vi "Start Async.vi"(8 "error in":errorcluster, 11 "gRPC Server in":refnum<class "ServiceBase.lvclass">) -> (0 "error out":errorcluster, 3 "gRPC Server out":refnum<class "ServiceBase.lvclass">)   [LabVIEW 2020, in "gRPC-servicer-release.lvlib" / "ServiceBase.lvclass"]
uses:
  gRPC Data Server Engine Windows.llb/ServiceBase.lvclass
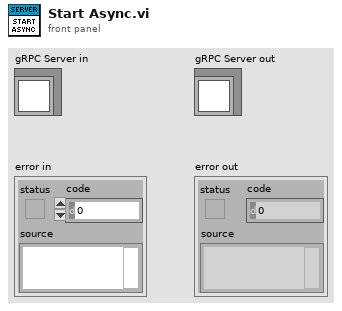
[diagram p1: front panel]
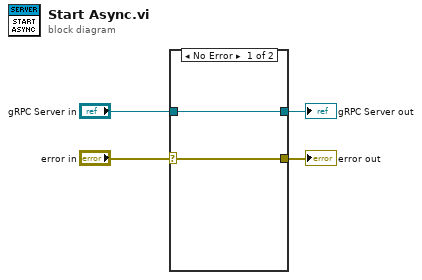
[diagram p0: block diagram]
diagram:
  n1 = case shown="No Error" "error in" {
    selector: "error in" -> [w6 w8]
    tunnel: [w6 w8] -> w3
    tunnel: [w5 w7] -> w1
    tunnel: "gRPC Server in" -> [w5 w7]
    frame No Error {
    }
    frame Error {
    }
  }
  "error out" <- w3
  "gRPC Server out" <- w1
